vi "Build ReadAdv.vi"(4 "ReadCfg":T1, 6 "Where":string, 8 "error in (no error)":errorcluster, 9 "tableName":string, 10 "DynamicParameters in":refnum<class "DynamicParameters.lvclass">, 11 "DbConnection in":refnum<class "DbConnection.lvclass">) -> (0 "error out":errorcluster, 2 "Query":string, 3 "DbConnection out":refnum<class "DbConnection.lvclass">)   [LabVIEW 2020, in "ORM.lvlib" / "DbConnection.lvclass"]
uses:
  DbConnection.lvclass
  DynamicParameters/DynamicParameters.lvclass
  AdvReadCfg.ctl
  OrderBy.ctl
  DbConnection.lvclass/DbConnection.ctl
  DynamicParameters/DynamicParameters.lvclass/DynamicParameters.ctl
  DynamicParameters/Read FieldNames.vi
  DynamicParameters/Read ParameterNames.vi
  Read ColumnNameEqualsValueFormat.vi
  <vilib>/regexp/Match Regular Expression.xnode
  ORM.lvlib
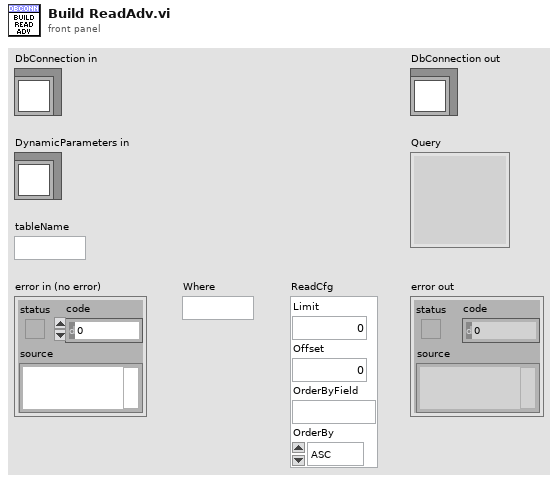
[diagram p1: front panel]
types:
  T1 = typedef "ORM.lvlib/AdvReadCfg.ctl" = cluster{"Limit":i64, "Offset":i64, "OrderByField":string, "OrderBy":T2}
  T2 = typedef "ORM.lvlib/OrderBy.ctl" = enum16{"ASC", "DESC"}
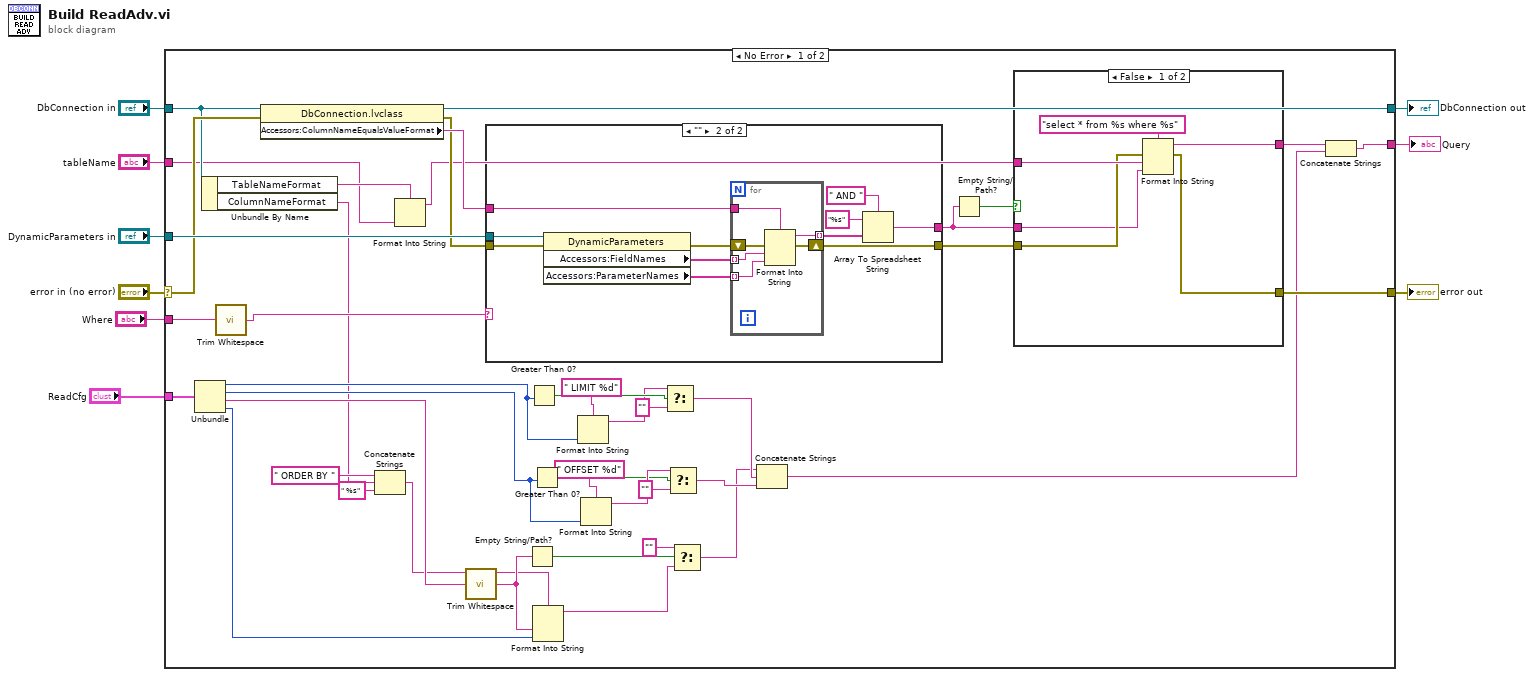
[diagram p0: block diagram]
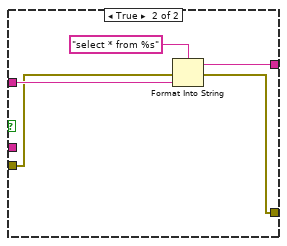
[diagram p2: hidden frame]
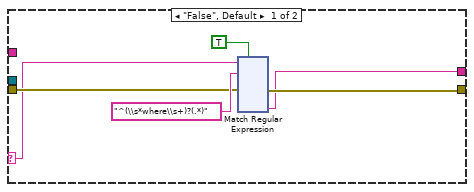
[diagram p3: hidden frame]
diagram:
  n1 = case shown="No Error" "error in (no error)" {
    selector: "error in (no error)" -> [w48 w204]
    tunnel: [w45 w204] -> w8
    tunnel: [w51 w203] -> w6
    tunnel: "DbConnection in" -> [w34 w203]
    tunnel: "DynamicParameters in" -> [w50 _]
    tunnel: "tableName" -> [w32 _]
    tunnel: [w35 _] -> w3
    tunnel: "Where" -> [w44 _]
    tunnel: "ReadCfg" -> [w26 _]
    frame No Error {
      n2 = Unbundle(w26) -> ("Limit"=w25:i64, "Offset"=w24:i64, "OrderByField"=w23:string, "OrderBy"=w21:T2)
      n3 = Unbundle By Name(w34) -> ("TableNameFormat"=w33:string, "ColumnNameFormat"=w12:string)
      n4 = call <vilib>:"Trim Whitespace.vi"("string"=w44) -> ("trimmed string"=w43:string)  [unwired: 1 in]
      n5 = property class="DbConnection.lvclass"(reference=w34, error in=w48) -> (reference out=w51:refnum<class "DbConnection.lvclass">, error out=w47:errorcluster, "Accessors:ColumnNameEqualsValueFormat"=w49:string)
      n6 = Concatenate Strings(" ORDER BY " ("format string"), w12, " %s" ("string")) -> (w10:string)
      n7 = Format Into String(format string=w33, w32) -> (resulting string=w31:string)  [unwired: 2 in, 1 out]
      n8 = call <vilib>:"Trim Whitespace.vi"("string"=w23) -> ("trimmed string"=w22:string)  [unwired: 1 in]
      n9 = case shown="\"\"" w43 {
        selector: w43 -> [w64 _]
        tunnel: w50 -> [_ w196]
        tunnel: w49 -> [_ w193]
        tunnel: [w63 w192] -> w42
        tunnel: w47 -> [w66 w188]
        tunnel: [w65 w186] -> w46
        frame "False", Default {
          n10 = xnode "Match Regular Expression"("input string"=w64, "regular expression"="^(\\s*where\\s+)?(.*)", "error in"=w66, "ignore case? (F)"=TRUE) -> ("error out"=w65:errorcluster, "submatch 2"=w63:string)  [unwired: 2 in, 5 out]
        }
        frame "" {
          n11 = property class="DynamicParameters"(reference=w196, error in=w188) -> (error out=w187:errorcluster, "Accessors:FieldNames"=w195:string[], "Accessors:ParameterNames"=w194:string[])  [unwired: 1 out]
          n12 = for {
            tunnel: w195 -> [w201] mode=indexing
            tunnel: w194 -> [w200] mode=indexing
            tunnel: w193 -> [w202]
            tunnel: [w199] -> w190 mode=indexing
            shift-right: [w197] -> w186
            shift-left: w187 -> [w198]
            n13 = Format Into String(format string=w202, error in=w198, w201, w200) -> (resulting string=w199:string, error out=w197:errorcluster)  [unwired: 1 in]
          }
          n14 = Array To Spreadsheet String(delimiter (Tab)=" AND ", array=w190, 3:"%s" ("format string")) -> (spreadsheet string=w192:string)
        }
      }
      n15 = Empty String/Path?(string/path=w22) -> (empty?=w20:bool)
      n16 = Greater Than 0?(x=w25) -> (x > 0?=w39:bool)
      n17 = Greater Than 0?(x=w24) -> (x > 0?=w28:bool)
      n18 = Format Into String(format string=w10, w22, w21) -> (resulting string=w19:string)  [unwired: 2 in, 1 out]
      n19 = Format Into String(format string=" LIMIT %d", w25) -> (resulting string=w38:string)  [unwired: 2 in, 1 out]
      n20 = Format Into String(format string=" OFFSET %d", w24) -> (resulting string=w29:string)  [unwired: 2 in, 1 out]
      n21 = Select(t=w38, s=w39, f="") -> (s? t:f=w17:string)
      n22 = Select(t=w29, s=w28, f="") -> (s? t:f=w16:string)
      n23 = Select(t="", s=w20, f=w19) -> (s? t:f=w15:string)
      n24 = Concatenate Strings(w15, w17, w16) -> (w14:string)
      n25 = Empty String/Path?(string/path=w42) -> (empty?=w41:bool)
      n26 = case shown="False" w41 {
        tunnel: w31 -> [w56 w61]
        tunnel: [w55 w59] -> w36
        tunnel: w46 -> [w54 w58]
        tunnel: [w53 w60] -> w45
        tunnel: w42 -> [w52 _]
        frame False {
          n27 = Format Into String(format string="select * from %s where %s", error in=w54, w56, w52) -> (resulting string=w55:string, error out=w53:errorcluster)  [unwired: 1 in]
        }
        frame True {
          n28 = Format Into String(format string="select * from %s", error in=w58, w61) -> (resulting string=w59:string, error out=w60:errorcluster)  [unwired: 1 in]
        }
      }
      n29 = Concatenate Strings(w36, w14) -> (w35:string)
    }
    frame Error {
    }
  }
  "error out" <- w8
  "DbConnection out" <- w6
  "Query" <- w3
